vi "test_speed.vi"() -> ()   [LabVIEW 2020]
panel:
  out "timestape":dbl format="%_19f"
  in  "stop":bool
  out "elapsed":dbl format="%0.2f"
  out "output array":dbl[][](array[numeric])
  in  "width & height":u16
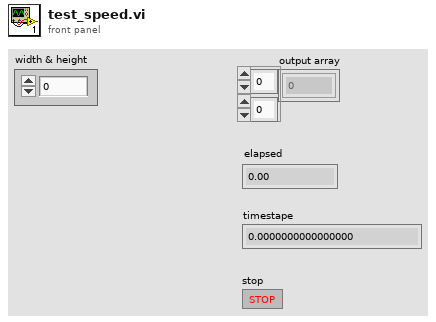
[diagram p1: front panel]
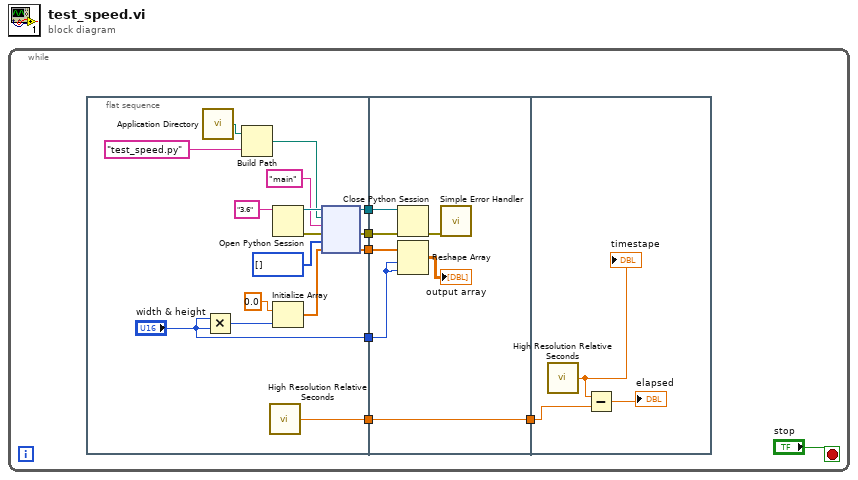
[diagram p0: block diagram]
diagram:
  n1 = while {
    stop <- "stop" stop-if-true
    n2 = flat-sequence {
      tunnel: [w15] -> w7
      tunnel: [w14] -> w6
      tunnel: [w13] -> w5
      tunnel: ["width & height"] -> w4
      tunnel: [w9] -> w2
      tunnel: w7 -> [w26]
      tunnel: w6 -> [w27]
      tunnel: w5 -> [w28]
      tunnel: w4 -> [w24]
      tunnel: [w25] -> w3
      tunnel: w2 -> [w25]
      tunnel: w3 -> [w32]
      frame #0 {
        n3 = call <vilib>:"Application Directory.vi"() -> ("Application Directory"=w23:path)
        n4 = Multiply(x="width & height", y="width & height") -> (x*y=w12:u16)
        n5 = Build Path(base path=w23, name or relative path="test_speed.py") -> (appended path=w20:path)
        n6 = call <vilib>:"High Resolution Relative Seconds.vi"() -> ("relative seconds"=w9:dbl)
        n7 = Open Python Session(python version="3.6") -> (session out=w21:refnum<k35>, error out=w22:errorcluster)  [unwired: 2 in]
        n8 = Initialize Array(0.0 ("element"), w12) -> (w10:dbl[])
        n9 = node(w21, w20, "main" ("함수 이름"), w22, u8[] [], w10) -> (w14:refnum<k35>, w15:errorcluster, w13:dbl[])  [unwired: 1 in, 2 out]
      }
      frame #1 {
        n10 = Close Python Session(session in=w27, error in=w26) -> (11:w29:errorcluster)
        n11 = Reshape Array(w28, w24, w24) -> (→"output array":dbl[][])
        n12 = call <vilib>:"Simple Error Handler.vi"("error in (no error)"=w29) -> ()  [unwired: 4 in, 5 out]
      }
      frame #2 {
        n13 = call <vilib>:"High Resolution Relative Seconds.vi"() -> ("relative seconds"=w33:dbl)
        "timestape" <- w33
        n14 = Subtract(x=w33, y=w32) -> (x-y=→"elapsed":dbl)
      }
    }
  }
